vi "solar_app Splash Close.vi"(8 "error in (no error)":errorcluster, 10 "Close Front Panel? (T)":bool=TRUE, 11 "Splash VI Refnum in":refnum<vi>) -> (0 "error out":errorcluster)   [LabVIEW 2018]
doc: "This closes the splash screen window."
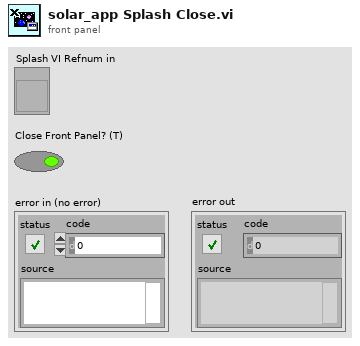
[diagram p1: front panel]
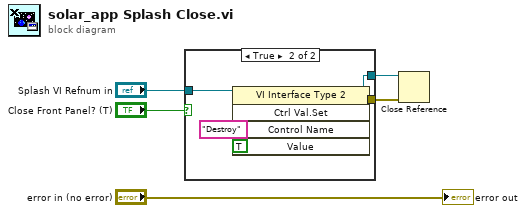
[diagram p0: block diagram]
diagram:
  n1 = case shown="True" "Close Front Panel? (T)" {
    tunnel: "Splash VI Refnum in" -> [w6 w11]
    tunnel: [_ w9] -> w4
    tunnel: [w6 w8] -> w3
    frame False {
    }
    frame True {
      n2 = invoke class="VI Interface Type 2" method="Ctrl Val.Set"(reference=w11, "Control Name"="Destroy", "Value"=TRUE) -> (reference out=w8:refnum<vi>, error out=w9:errorcluster)  [unwired: 2 in, 3 out]
    }
  }
  n3 = Close Reference(reference=w3, error in (no error)=w4) -> ()  [unwired: 1 out]
  "error out" <- "error in (no error)"
